vi "MovAvg.vi"(11 "Array in":dbl[](array[numeric])) -> (3 "Array out":dbl[](array[numeric]))   [LabVIEW 2020]
doc: "Esta funcion Genera un calculo del promedio movil de una señal (Tamaño de ventana fijo = 6)"
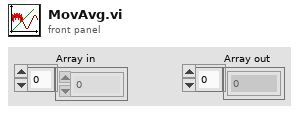
[diagram p1: front panel]
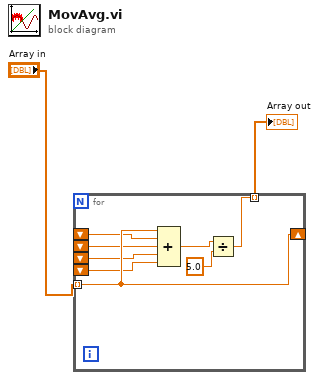
[diagram p0: block diagram]
diagram:
  n1 = for {
    tunnel: "Array in" -> [w10] mode=indexing
    shift-right: [w10] -> _
    shift-left: _ -> [w9]
    shift-left: _ -> [w8]
    shift-left: _ -> [w7]
    shift-left: _ -> [w6]
    tunnel: [w3] -> w2 mode=indexing
    n2 = Compound Arithmetic op=ADD(w10, w9, w8, w7, w6) -> (w5:dbl)
    n3 = Divide(x=w5, y=5.0) -> (x/y=w3:dbl)
  }
  "Array out" <- w2
